vi "Read.vi"(8 "error in (no error)":errorcluster, 10 "count":i32, 11 "File Upload Controller in":refnum<class "File Upload Controller.lvclass">) -> (0 "error out":errorcluster, 2 "data":u8[](array[numeric]), 3 "File Upload Controller out":refnum<class "File Upload Controller.lvclass">)   [LabVIEW 2020, in "NI_SFTP.lvlib" / "File Upload Controller.lvclass"]
uses:
  <vilib>/net/SFTP/API/Support/Upload/File/File Upload Controller.lvclass
  <vilib>/net/SFTP/API/Support/Upload/File/File Upload Controller.lvclass/File Upload Controller.ctl
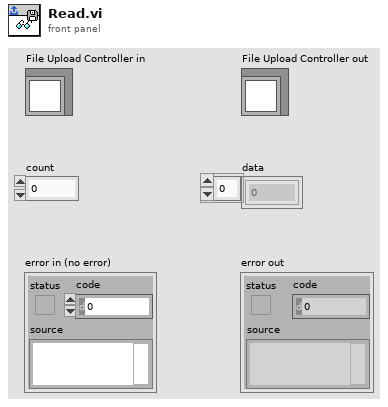
[diagram p1: front panel]
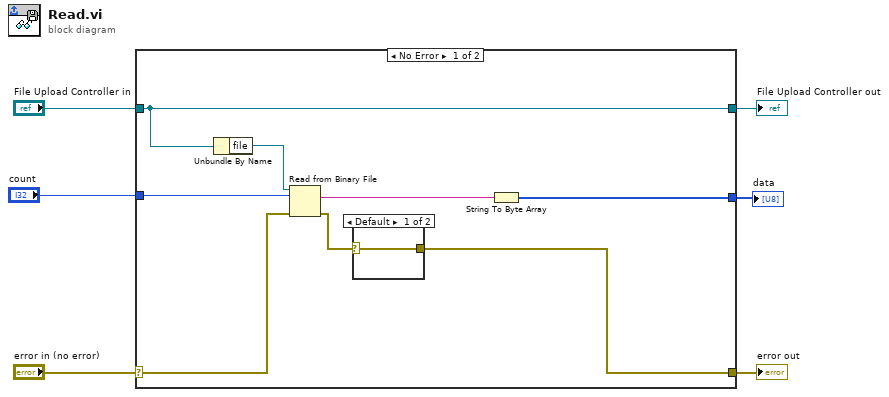
[diagram p0: block diagram]
diagram:
  n1 = case shown="No Error" "error in (no error)" {
    selector: "error in (no error)" -> [w11 w17]
    tunnel: [w7 w17] -> w5
    tunnel: [w14 w16] -> w3
    tunnel: "File Upload Controller in" -> [w14 w16]
    tunnel: "count" -> [w12 _]
    tunnel: [w9 _] -> w1
    frame No Error {
      n2 = Unbundle By Name(w14) -> ("file"=w13:refnum<file>)
      n3 = Read from Binary File(8:w11, 10:w12, 11:w13) -> (0:w8:errorcluster, 2:w10:string)  [unwired: 3 in, 2 out]
      n4 = case shown="Default" w8 {
        selector: w8 -> [w15 _]
        tunnel: [w15 _] -> w7
        frame #0 {
        }
        frame #1 {
        }
      }
      n5 = String To Byte Array(string=w10) -> (unsigned byte array=w9:u8[])
    }
    frame Error {
    }
  }
  "error out" <- w5
  "File Upload Controller out" <- w3
  "data" <- w1
